vi "DDS9959 Set Frequency.vi"(0 "VISA resource name":refnum<visa-resource-name>, 1 "Register":string(combo)="04", 5 "Set Frequency (MHz)":dbl format="%#_10g", 7 "Channel":u16=1 min=1 max=4, 9 "Clock Frequency (MHz)":dbl, 11 "error in (no error)":errorcluster) -> (4 "VISA resource name out":refnum<visa-resource-name>, 15 "error out":errorcluster)   [LabVIEW 2012]
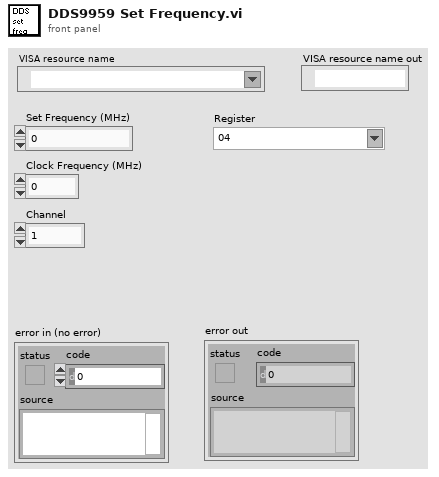
[diagram p1: front panel]
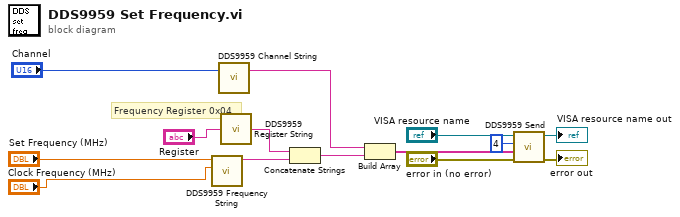
[diagram p0: block diagram]
diagram:
  # "Frequency Register 0x04"
  n1 = call "DDS9959 Frequency String.vi"("Clock Frequency (MHz)"="Clock Frequency (MHz)", "Set Frequency (MHz)"="Set Frequency (MHz)") -> ("String"=w14:string)  [unwired: 9 in]
  n2 = call "DDS9959 Channel String.vi"("Channel"="Channel") -> ("String"=w1:string)  [unwired: 2 in]
  n3 = call "DDS9959 Register String.vi"("register"="Register") -> ("output"=w3:string)
  n4 = Concatenate Strings(w3, w14) -> (w13:string)
  n5 = Build Array(w1, w13) -> (w12:string[])
  n6 = call "DDS9959 Send.vi"("error in (no error)"="error in (no error)", "Output Array"=w12, "USB Out Endpoint"=i16 4, "VISA resource name"="VISA resource name") -> ("error out"=→"error out":errorcluster, "VISA resource name"=→"VISA resource name out":refnum<visa-resource-name>)  [unwired: 6 in]
